vi "Hyperslab Blocks to Pointlist.vi"(1 "Hyperslab Blocks":cluster{"Start":u64[], "Opposite":u64[]}[](array[cluster])) -> (0 "Pointlist":u64[][](array[numeric]))   [LabVIEW 2017]
panel:
  # "LVHDF5 Toolkit\nCopyright (c) 2005-2013 by Jason D. Sommerville\nCopyright (c) 2014 by UPVI, LLC.\n\nThis use and distribution of this file is governed by the terms found in \nLICENSE.txt distributed with this toolkit and installed at\n <user.lib>\\_lvhdf5\\LICENSE.txt"
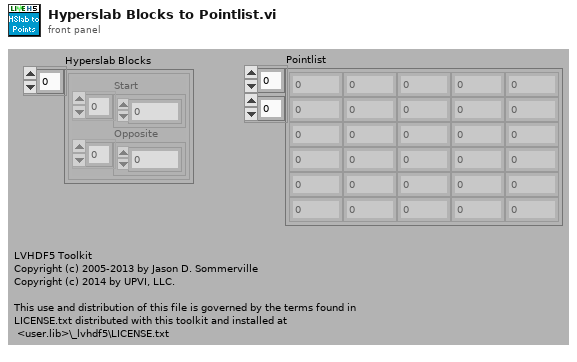
[diagram p1: front panel]
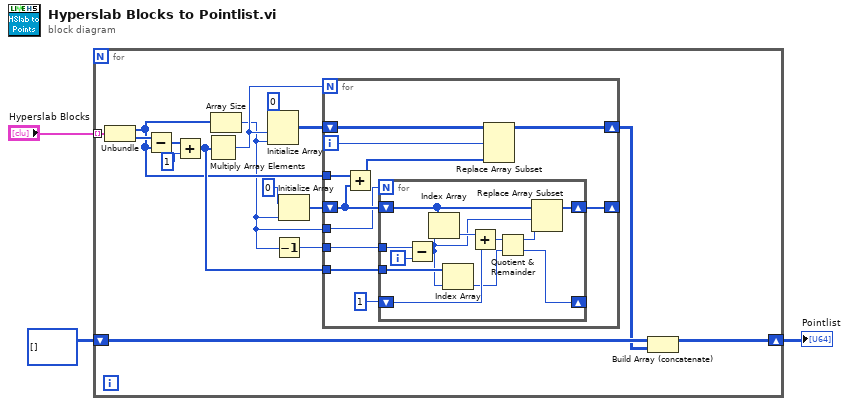
[diagram p0: block diagram]
diagram:
  n1 = for {
    tunnel: "Hyperslab Blocks" -> [w19] mode=indexing
    shift-right: [w15] -> w1
    shift-left: u64[][] [] -> [w14]
    n2 = Unbundle(w19) -> ("Start"=w8:u64[], "Opposite"=w18:u64[])
    n3 = Subtract(x=w18, y=w8) -> (x-y=w17:u64[])
    n4 = Add(x=w17, y=1) -> (x+y=w10:u64[])
    n5 = Multiply Array Elements(1:w10) -> (0:w9:u64)
    n6 = Array Size(array=w8) -> (size(s)=w4:i32)
    n7 = Initialize Array(u32 0, w9, w4) -> (w12:u32[][])
    n8 = Decrement(x=w4) -> (x-1=w5:i32)
    n9 = Initialize Array(u32 0, w4) -> (w6:u32[])
    n10 = for {
      N: w9 -> [_]
      shift-right: [w29] -> w11
      shift-left: w12 -> [w30]
      tunnel: w10 -> [w27]
      shift-right: [w26] -> _
      shift-left: w6 -> [w24]
      tunnel: w8 -> [w25]
      tunnel: w5 -> [w21]
      tunnel: w4 -> [w20]
      i -> [w28]
      n11 = Add(x=w25, y=w24) -> (x+y=w23:u64[])
      n12 = for {
        N: w20 -> [_]
        tunnel: w27 -> [w33]
        shift-right: [w37] -> _
        shift-left: u32 1 -> [w34]
        shift-right: [w38] -> w26
        shift-left: w24 -> [w40]
        tunnel: w21 -> [w42]
        i -> [w41]
        n13 = Subtract(x=w42, y=w41) -> (x-y=w32:i32)
        n14 = Index Array(array=w40, index=w32) -> (element=w35:u32)
        n15 = Index Array(array=w33, index=w32) -> (element=w31:u64)
        n16 = Add(x=w35, y=w34) -> (x+y=w36:u64)
        n17 = Quotient & Remainder(x=w36, y=w31) -> (x-y*floor(x/y)=w39:u64, floor(x/y)=w37:u64)
        n18 = Replace Array Subset(array=w40, new element=w39, index=w32) -> (w38:u32[])
      }
      n19 = Replace Array Subset(array=w30, new element=w23, index (row)=w28) -> (w29:u32[][])  [unwired: 1 in]
    }
    n20 = Build Array (concatenate)(w14, w11) -> (w15:u64[][])
  }
  "Pointlist" <- w1
